vi "From Value.vi"(8 "error in (no error)":errorcluster, 10 "PV Data in":refnum<class "PV Data.lvclass">, 11 "NT Base in":refnum<class "NT Base.lvclass">) -> (0 "error out":errorcluster, 2 "PV Data out":refnum<class "PV Data.lvclass">, 3 "NT Base out":refnum<class "NT Base.lvclass">)   [LabVIEW 2020, in "PV Access.lvlib" / "PV Data.lvlib" / "NT Base.lvclass"]
uses:
  NT Base.lvclass
  NT Base.lvclass/NT Base.ctl
  PV Data/PV Data.lvclass
  PV Data/Read Field (Variant).vi
  PV Data/Read Field (String).vi
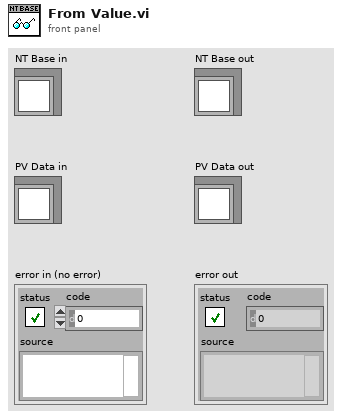
[diagram p1: front panel]
types:
  T1 = typedef "PV Access.lvlib/PV Data.lvlib/Alarm.ctl" = cluster{"Severity":T2, "Status":T3, "Message":string}
  T2 = typedef "PV Access.lvlib/PV Data.lvlib/Alarm Severity.ctl" = enum32{"no", "minor", "major", "record", "invalid", "undefined", ""}
  T3 = typedef "PV Access.lvlib/PV Data.lvlib/Alarm Status.ctl" = enum32{"no", "device", "driver", "record", "db", "conf", "undefined", "client"}
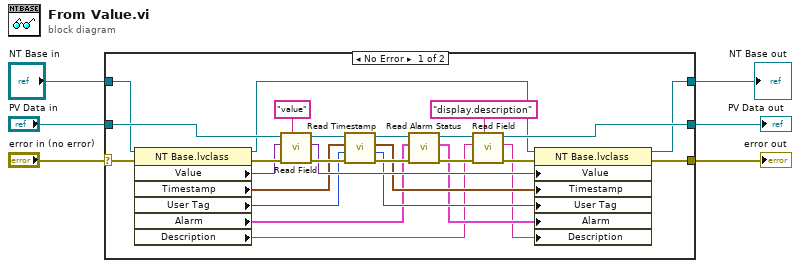
[diagram p0: block diagram]
diagram:
  n1 = case shown="No Error" "error in (no error)" {
    selector: "error in (no error)" -> [w28 w36]
    tunnel: [w25 w36] -> w5
    tunnel: [w24 w35] -> w3
    tunnel: "NT Base in" -> [w27 w35]
    tunnel: [w30 w34] -> w1
    tunnel: "PV Data in" -> [w33 w34]
    frame No Error {
      n2 = property class="NT Base.lvclass"(reference=w27, error in=w28) -> (reference out=w23:refnum<class "NT Base.lvclass">, error out=w29:errorcluster, "Value"=w16:variant, "Timestamp"=w14:timestamp, "User Tag"=w13:i32, "Alarm"=w10:T1, "Description"=w8:string)
      n3 = call-poly "Read Field.vi"("field name"="value", "error in (no error)"=w29, "value"=w16, "PV Data in"=w33) -> ("error out"=w22:errorcluster, "value out"=w15:variant, "PV Data out"=w19:refnum<class "PV Data.lvclass">)  [unwired: 4 in, 1 out]
      n4 = call "Read Timestamp.vi"("error in"=w22, "user tag in"=w13, "timestamp in"=w14, "PV Data in"=w19) -> ("error out"=w21:errorcluster, "user tag"=w11:i32, "timestamp"=w12:timestamp, "PV Data out"=w18:refnum<class "PV Data.lvclass">)  [unwired: 4 in]
      n5 = call "Read Alarm Status.vi"("error in"=w21, "alarm status in"=w10, "PV Data in"=w18) -> ("error out"=w20:errorcluster, "alarm status out"=w9:T1, "PV Data out"=w17:refnum<class "PV Data.lvclass">)  [unwired: 5 in, 1 out]
      n6 = call-poly "Read Field.vi"("field name"="display.description", "error in (no error)"=w20, "default"=w8, "PV Data in"=w17) -> ("error out"=w26:errorcluster, "value"=w7:string, "PV Data out"=w30:refnum<class "PV Data.lvclass">)  [unwired: 5 in]
      n7 = property class="NT Base.lvclass"(reference=w23, error in=w26, "Value"=w15, "Timestamp"=w12, "User Tag"=w11, "Alarm"=w9, "Description"=w7) -> (reference out=w24:refnum<class "NT Base.lvclass">, error out=w25:errorcluster)
    }
    frame Error {
    }
  }
  "error out" <- w5
  "NT Base out" <- w3
  "PV Data out" <- w1
